vi "Connect AutoLab.vi"(10 "Embedded Exe File":path=path "C:/Users/Benj/Desktop/Autolab software stuff/Minimal working example/Adk.x", 11 "Hardware Setup File":path=path "C:/Users/Benj/Desktop/Autolab software stuff/Minimal working example/HardwareSetup.AUT55157.xml") -> (0 "error out":errorcluster, 3 ".NET Refnum out":refnum<k24>)   [LabVIEW 2022 SP3]
uses:
  C:/Users/Benj/Desktop/SEC Software V4.9/EcoChemie.Autolab.Sdk.dll
  EcoChemie.Autolab.Sdk.dll
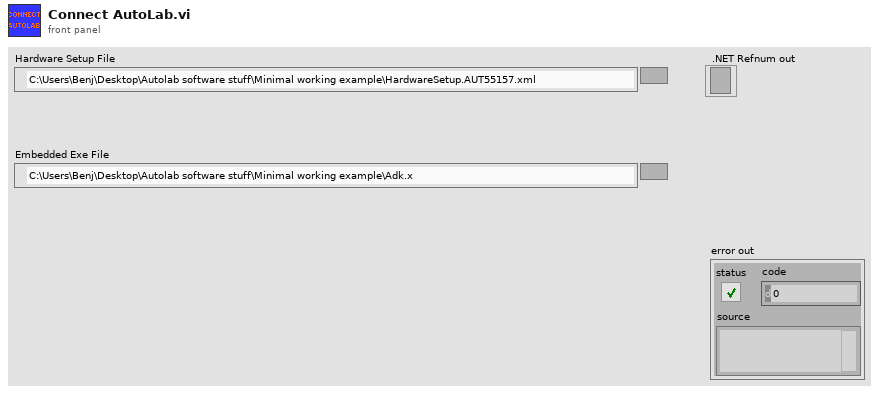
[diagram p1: front panel]
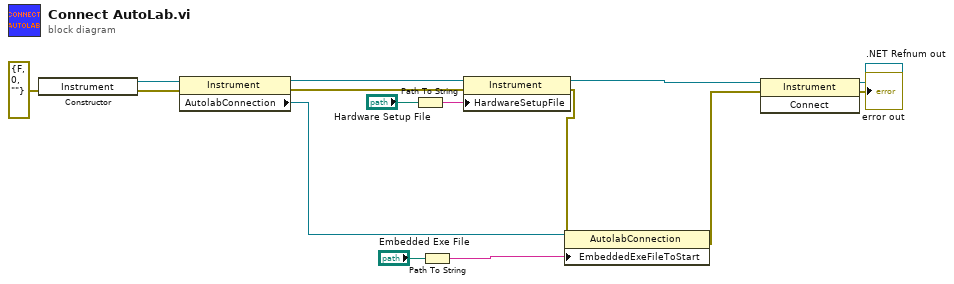
[diagram p0: block diagram]
diagram:
  n1 = constructor class="Instrument"(error in=errorcluster {"status"=FALSE, "code"=0, "source"=""} ("error in (no error)")) -> (reference out=w7:refnum<k24>, error out=w1:errorcluster)  [unwired: 2 in, 1 out]
  n2 = property class="Instrument"(reference=w7, error in=w1) -> (reference out=w8:refnum<k24>, error out=w9:errorcluster, "AutolabConnection"=w3:refnum<k24>)
  n3 = Path To String(path="Hardware Setup File") -> (string=w5:string)
  n4 = Path To String(path="Embedded Exe File") -> (string=w10:string)
  n5 = property class="Instrument"(reference=w8, error in=w9, "HardwareSetupFile"=w5) -> (reference out=w13:refnum<k24>, error out=w11:errorcluster)
  n6 = property class="AutolabConnection"(reference=w3, error in=w11, "EmbeddedExeFileToStart"=w10) -> (error out=w12:errorcluster)  [unwired: 1 out]
  n7 = invoke class="Instrument" method="Connect"(reference=w13, error in=w12) -> (reference out=→".NET Refnum out":refnum<k24>, error out=→"error out":errorcluster)  [unwired: 1 in, 1 out]
